vi "模拟输入_连续.vi"() -> ()   [LabVIEW 2013]
doc: "This example demonstrates how to acquire a continuous data."
uses:
  <userlib>/ArtDAQ/_SubVI/ArtDAQ_CreateAIVoltageChan.vi
  <userlib>/ArtDAQ/_SubVI/ArtDAQ_CfgSampClkTiming.vi
  <userlib>/ArtDAQ/_SubVI/ArtDAQ_CfgDigEdgeStartTrig.vi
  <userlib>/ArtDAQ/_SubVI/ArtDAQ_CfgAnlgEdgeStartTrig.vi
  <userlib>/ArtDAQ/_SubVI/ArtDAQ_CfgAnlgWindowStartTrig.vi
  <userlib>/ArtDAQ/_SubVI/ArtDAQ_Read Analog DBL NChan NSamp.vi
panel:
  in  "触发模式":enum32{"无触发", "数字边沿", "模拟边沿", "模拟窗"}(tab)
  in  "触发源":string="/Dev1/PFI1"
  in  "触发边沿":i32(ring)=10280 items=["上升"=10280, "下降"=10171]
  in  "触发电平(V)":dbl
  in  "触发源":string(combo)="Dev1/ai0"
  in  "斜率":i32(ring)=10280 items=["上升"=10280, "下降"=10171]
  in  "触发条件":i32(ring)=10163 items=["进入窗"=10163, "离开窗"=10208]
  in  "窗顶部":dbl=0.5
  in  "窗底部":dbl
  in  "触发源":string(combo)="Dev1/ai0"
  in  "停止":bool
  out "Waveform":dbl[][](graph)
  in  "采样频率":dbl=10000.0 format="%#_13g"
  in  "每通道采样点数":i32=1000
  in  "接地方式":i32(ring)=10083 items=["默认"=-1, "单端"=10083, "非参考单端"=10078, "差分"=10106, "伪差分"=12529]
  in  "最小值(V)":dbl=-10.0 format="%#_13g"
  in  "最大值(V)":dbl=10.0 format="%#_13g"
  in  "物理通道":string(combo)="Dev1/ai0"
  out "错误":errorcluster
  # "通道属性"
  # "定时"
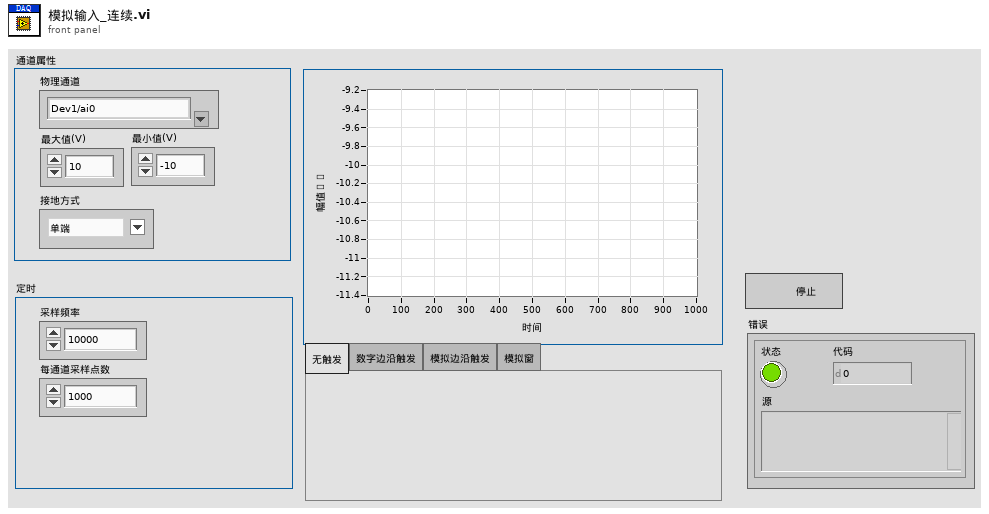
[diagram p1: front panel]
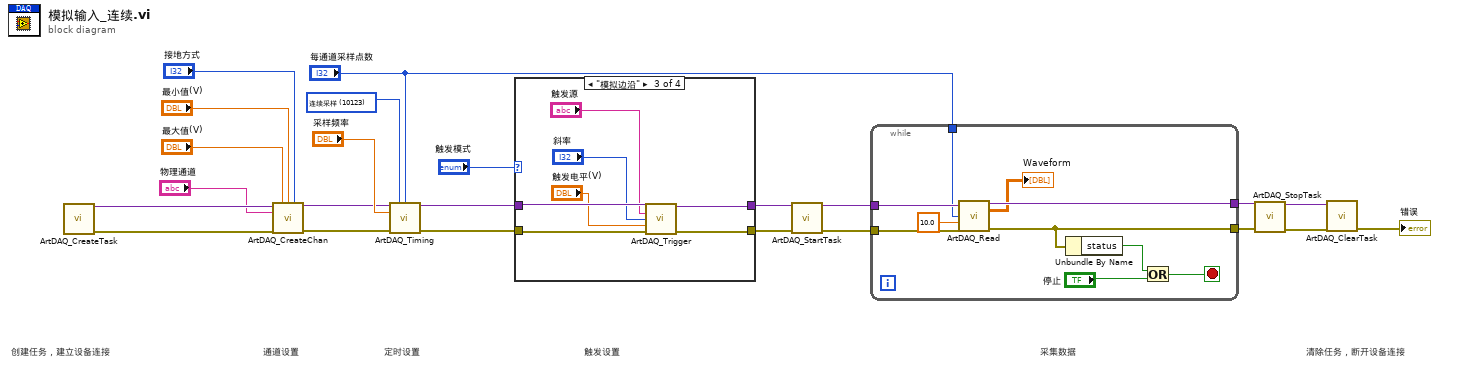
[diagram p0: block diagram]
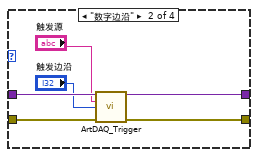
[diagram p3: hidden frame]
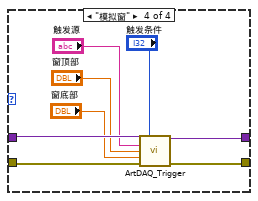
[diagram p4: hidden frame]
diagram:
  w1 = 10123 items=["有限点采样"=10178, "连续采样"=10123] ("SampleMode")
  # "清除任务，断开设备连接"
  # "采集数据"
  # "触发设置"
  # "定时设置"
  # "通道设置"
  # "创建任务，建立设备连接"
  n1 = call <userlib>:"ArtDAQ_CreateTask.vi"() -> ("任务句柄"=w13:variant, "错误输出"=w23:errorcluster)  [unwired: 14 in]
  n2 = call-poly <userlib>:"ArtDAQ_CreateChan.vi"("任务句柄"=w13, "最大值"="最大值(V)", "最小值"="最小值(V)", "接线端配置"="接地方式", "物理通道"="物理通道", "错误输入"=w23) -> ("任务句柄"=w2:variant, "错误输出"=w19:errorcluster)  [unwired: 8 in]
  n3 = call-poly <userlib>:"ArtDAQ_Timing.vi"("任务句柄"=w2, "采样模式"=w1, "每通道采样数"="每通道采样点数", "采样率"="采样频率", "错误输入"=w19) -> ("任务句柄"=w7:variant, "错误输出"=w5:errorcluster)  [unwired: 9 in]
  n4 = case shown="\"模拟边沿\"" "触发模式" {
    tunnel: w7 -> [w25 w31 w38 w46]
    tunnel: [w25 w30 w37 w45] -> w6
    tunnel: w5 -> [w24 w28 w35 w43]
    tunnel: [w24 w29 w36 w44] -> w4
    frame "无触发", Default {
    }
    frame "数字边沿" {
      n5 = call-poly <userlib>:"ArtDAQ_Trigger.vi"("任务句柄"=w31, "触发源"="触发源", "边沿"="触发边沿", "错误输入"=w28) -> ("任务句柄"=w30:variant, "错误输出"=w29:errorcluster)  [unwired: 10 in]
    }
    frame "模拟边沿" {
      n6 = call-poly <userlib>:"ArtDAQ_Trigger.vi"("任务句柄"=w38, "触发源"="触发源", "斜率"="斜率", "触发电平"="触发电平(V)", "错误输入"=w35) -> ("任务句柄"=w37:variant, "错误输出"=w36:errorcluster)  [unwired: 9 in]
    }
    frame "模拟窗" {
      n7 = call-poly <userlib>:"ArtDAQ_Trigger.vi"("任务句柄"=w46, "触发条件"="触发条件", "触发源"="触发源", "窗顶部"="窗顶部", "窗底部"="窗底部", "错误输入"=w43) -> ("任务句柄"=w45:variant, "错误输出"=w44:errorcluster)  [unwired: 8 in]
    }
  }
  n8 = call <userlib>:"ArtDAQ_StartTask.vi"("任务句柄"=w6, "错误输入"=w4) -> ("任务句柄"=w16:variant, "错误输出"=w15:errorcluster)  [unwired: 12 in]
  n9 = while {
    tunnel: w16 -> [w56]
    tunnel: w15 -> [w55]
    tunnel: "每通道采样点数" -> [w54]
    tunnel: [w52] -> w12
    tunnel: [w51] -> w11
    stop <- w49 stop-if-true
    n10 = call-poly <userlib>:"ArtDAQ_Read.vi"("任务句柄"=w56, "每通道采样数"=w54, "超时s"=10.0 ("Timeout"), "错误输入"=w55) -> ("任务句柄"=w52:variant, "数据"=→"Waveform":dbl[][], "错误输出"=w51:errorcluster)  [unwired: 8 in, 1 out]
    n11 = Unbundle By Name(w51) -> ("status"=w50:bool)
    n12 = Or(x=w50, y="停止") -> (x .or. y?=w49:bool)
  }
  n13 = call <userlib>:"ArtDAQ_StopTask.vi"("任务句柄"=w12, "错误输入"=w11) -> ("任务句柄"=w10:variant, "错误输出"=w9:errorcluster)  [unwired: 12 in]
  n14 = call <userlib>:"ArtDAQ_ClearTask.vi"("任务句柄"=w10, "错误输入"=w9) -> ("错误输出"=→"错误":errorcluster)  [unwired: 13 in]
